vi "IntakeForTime.vi"() -> ()   [LabVIEW 2018]
uses:
  Framework/Robot Global Data.vi
panel:
  in  "NoWait":bool
  in  "Speed":dbl
  in  "Time":dbl
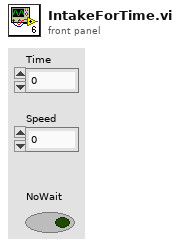
[diagram p1: front panel]
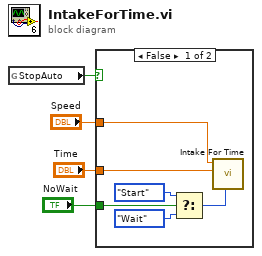
[diagram p0: block diagram]
diagram:
  n1 = global read "Robot Global Data.vi" "StopAuto"() -> (w4:bool)
  n2 = case shown="False" w4 {
    tunnel: "Time" -> [w6 _]
    tunnel: "Speed" -> [w7 _]
    tunnel: "NoWait" -> [w10 _]
    frame False {
      n3 = Select(t=enum16{"Start", "Wait"}."Start" ("Synchronization"), s=w10, f=enum16{"Start", "Wait"}."Wait" ("Synchronization")) -> (s? t:f=w5:enum16{"Start", "Wait"})
      n4 = call "Intake For Time.vi"("Synchronization"=w5, "Duration (s)"=w6, "Speed"=w7) -> ()  [unwired: 8 in, 1 out]
    }
    frame True {
    }
  }
